vi "Prepare Image For GIF.vi"(8 "error in (no error)":errorcluster, 11 "Image":T1) -> (0 "error out":errorcluster, 3 "Image":T1)   [LabVIEW 2020, in "G-Image.lvlib"]
uses:
  G-Image.lvlib
  <vilib>/picture/picture.llb/imagedata.ctl
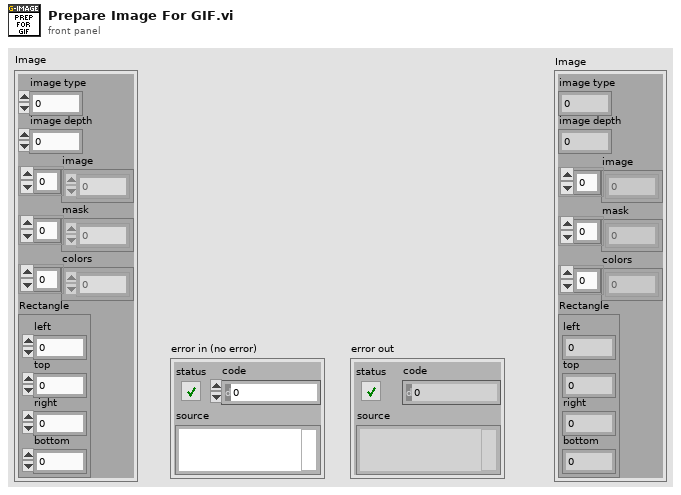
[diagram p1: front panel]
types:
  T1 = typedef "imagedata.ctl" = cluster{"image type":i32, "image depth":i32, "image":u8[], "mask":u8[], "colors":u32[], "Rectangle":cluster{"left":i16, "top":i16, "right":i16, "bottom":i16}}
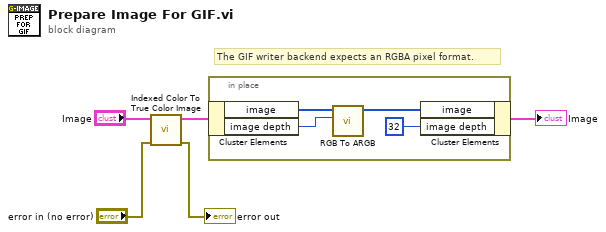
[diagram p0: block diagram]
diagram:
  # "The GIF writer backend expects an RGBA pixel format."
  n1 = call "Indexed Color To True Color Image.vi"("error in (no error)"="error in (no error)", "Indexed Image"="Image") -> ("error out"=→"error out":errorcluster, "True Color Image"=w5:T1)  [unwired: 8 in]
  n2 = in-place {
    n3 = in-place-cluster #1(w5) -> ("image"=w9:u8[], "image depth"=w8:i32)
    n4 = call "RGB To ARGB.vi"("Depth"=w8, "Image Data"=w9) -> ("RGBA"=w7:u8[])  [unwired: 9 in]
    n5 = in-place-cluster #1("image"=w7, "image depth"=32) -> (→"Image":T1)
  }
